vi "IncrementArrayByIndex.vi"(10 "index":i32, 11 "Array in":i32[](array[numeric])) -> (3 "Array out":i32[](array[numeric]))   [LabVIEW 2016]
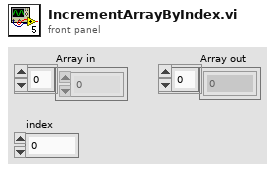
[diagram p1: front panel]
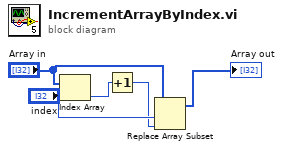
[diagram p0: block diagram]
diagram:
  n1 = Index Array(array="Array in", index="index") -> (element=w2:i32)
  n2 = Increment(x=w2) -> (x+1=w1:i32)
  n3 = Replace Array Subset(array="Array in", new element=w1, index="index") -> (→"Array out":i32[])
